vi "contet help.vi"() -> ()   [LabVIEW 2009]
uses:
  <vilib>/Utility/miscctls.llb/LVPointTypeDef.ctl
panel:
  in  "stop":bool
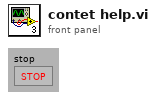
[diagram p1: front panel]
types:
  T1 = typedef "LVPointTypeDef.ctl" = cluster{"Horizontal":i16, "Vertical":i16}
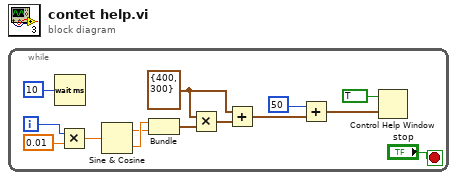
[diagram p0: block diagram]
diagram:
  n1 = while {
    i -> [w13]
    stop <- "stop" stop-if-true
    w4 = T1 {"Horizontal"=400, "Vertical"=300} ("Top Left Corner")
    n2 = Wait (ms)(milliseconds to wait=u32 10) -> ()  [unwired: 1 out]
    n3 = Multiply(x=w13, y=0.01) -> (x*y=w11:dbl)
    n4 = Sine & Cosine(0:w11) -> (1:w9:dbl, 2:w10:dbl)
    n5 = Bundle(w10, w9) -> (w8:cluster{dbl, dbl})  [unwired: 1 in]
    n6 = Multiply(x=w4, y=w8) -> (x*y=w7:cluster{dbl, dbl})
    n7 = Add(x=w4, y=w7) -> (x+y=w3:cluster{dbl, dbl})
    n8 = Add(x=50, y=w3) -> (x+y=w1:cluster{dbl, dbl})
    n9 = Control Help Window(0:w1, 1:TRUE ("Show")) -> ()
  }
